vi "convertTableToArray.vi"(8 "error in":errorcluster, 11 "tbl":string[][](array[string])) -> (0 "error out":errorcluster, 3 "contArr":string[](array[string]))   [LabVIEW 2010]
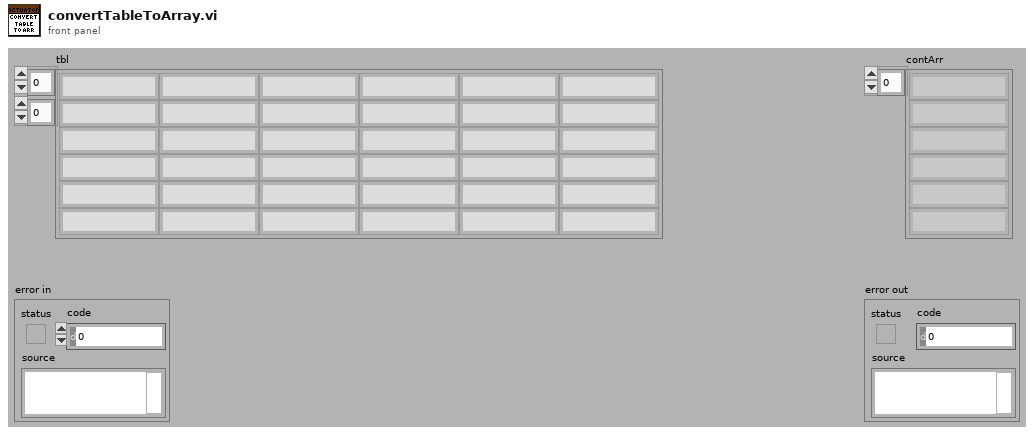
[diagram p1: front panel]
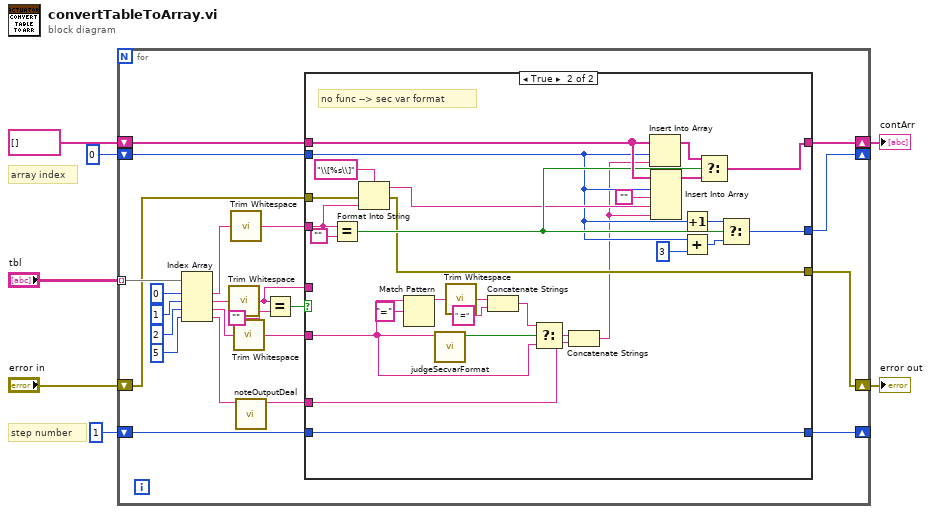
[diagram p0: block diagram]
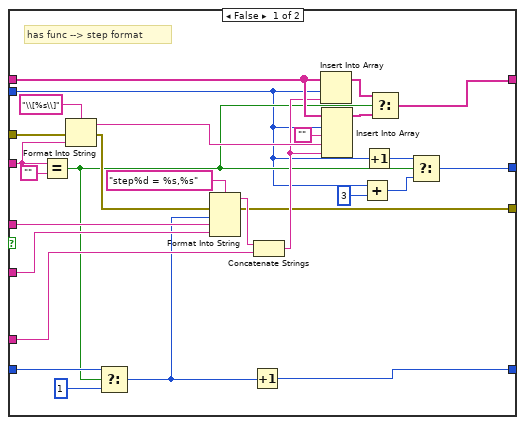
[diagram p2: hidden frame]
diagram:
  # "step number"
  # "array index"
  n1 = for {
    tunnel: "tbl" -> [w29] mode=indexing
    shift-right: [w11] -> w2
    shift-left: string[] [] ("Value") -> [w14]
    shift-right: [w8] -> w1
    shift-left: "error in" -> [w9]
    shift-right: [w10] -> _
    shift-left: 0 ("input 1") -> [w13]
    shift-right: [w12] -> _
    shift-left: 1 ("input 1") -> [w21]
    n2 = Index Array(array=w29, index #1=0 ("index"), index #2=1 ("index"), index #3=2 ("index"), index #4=5 ("index")) -> (element #1=w22:string, element #2=w25:string, element #3=w19:string, element #4=w16:string)
    n3 = call <vilib>:"Trim Whitespace.vi"("string"=w25) -> ("trimmed string"=w20:string)  [unwired: 1 in]
    n4 = call <vilib>:"Trim Whitespace.vi"("string"=w22) -> ("trimmed string"=w17:string)  [unwired: 1 in]
    n5 = call <vilib>:"Trim Whitespace.vi"("string"=w19) -> ("trimmed string"=w18:string)  [unwired: 1 in]
    n6 = call "noteOutputDeal.vi"("note in editor"=w16) -> ("note output"=w15:string)  [unwired: 10 in]
    n7 = Equal?(x=w20, y="") -> (x = y?=w23:bool)
    n8 = case shown="True" w23 {
      tunnel: w21 -> [w43 w60]
      tunnel: w20 -> [w56 _]
      tunnel: w18 -> [w55 w73]
      tunnel: w17 -> [w50 w83]
      tunnel: w15 -> [w53 w71]
      tunnel: w14 -> [w48 w80]
      tunnel: w13 -> [w36 w64]
      tunnel: [w40 w60] -> w12
      tunnel: [w34 w67] -> w11
      tunnel: [w33 w62] -> w10
      tunnel: w9 -> [w32 w84]
      tunnel: [w31 w61] -> w8
      frame False {
        # "has func --> step format"
        n9 = Equal?(x=w50, y="") -> (x = y?=w39:bool)
        n10 = Format Into String(format string="\\[%s\\]", error in=w32, w50) -> (resulting string=w46:string, error out=w49:errorcluster)  [unwired: 1 in]
        n11 = Select(t=w43, s=w39, f=1) -> (s? t:f=w41:i32)
        n12 = Format Into String(format string="step%d = %s,%s", error in=w49, w41, w56, w55) -> (resulting string=w54:string, error out=w31:errorcluster)  [unwired: 1 in]
        n13 = Increment(x=w41) -> (x+1=w40:i32)
        n14 = Concatenate Strings(w54, w53) -> (w45:string)
        n15 = Insert Into Array(array=w48, index=w36, new element=w45) -> (w52:string[])
        n16 = Insert Into Array(array=w48, index=w36, new element #1="", new element #2=w46, new element #3=w45) -> (w44:string[])
        n17 = Add(x=w36, y=3) -> (x+y=w37:i32)
        n18 = Increment(x=w36) -> (x+1=w38:i32)
        n19 = Select(t=w52, s=w39, f=w44) -> (s? t:f=w34:string[])
        n20 = Select(t=w38, s=w39, f=w37) -> (s? t:f=w33:i32)
      }
      frame True {
        # "no func --> sec var format"
        n21 = Equal?(x=w83, y="") -> (x = y?=w70:bool)
        n22 = Format Into String(format string="\\[%s\\]", error in=w84, w83) -> (resulting string=w68:string, error out=w61:errorcluster)  [unwired: 1 in]
        n23 = Match Pattern(string=w73, regular expression="=") -> (before substring=w77:string)  [unwired: 1 in, 3 out]
        n24 = call "judgeSecvarFormat.vi"("section variable"=w73) -> ("correct format?"=w79:bool)  [unwired: 10 in]
        n25 = call <vilib>:"Trim Whitespace.vi"("string"=w77) -> ("trimmed string"=w76:string)  [unwired: 1 in]
        n26 = Concatenate Strings(w76, " =" ("format string")) -> (w74:string)
        n27 = Select(t=w74, s=w79, f=w73) -> (s? t:f=w72:string)
        n28 = Concatenate Strings(w72, w71) -> (w59:string)
        n29 = Insert Into Array(array=w80, index=w64, new element=w59) -> (w82:string[])
        n30 = Insert Into Array(array=w80, index=w64, new element #1="", new element #2=w68, new element #3=w59) -> (w81:string[])
        n31 = Increment(x=w64) -> (x+1=w66:i32)
        n32 = Add(x=w64, y=3) -> (x+y=w63:i32)
        n33 = Select(t=w82, s=w70, f=w81) -> (s? t:f=w67:string[])
        n34 = Select(t=w66, s=w70, f=w63) -> (s? t:f=w62:i32)
      }
    }
  }
  "contArr" <- w2
  "error out" <- w1
